vi "Seg1_Charging_Limit_Voltage_checking.vi"(8 "error in (no error)":errorcluster, 9 "Numeric":i32, 10 "Stop Voltage(V)":dbl=4.34 format="%_3f", 11 "VISA Refnum in":refnum<visa-resource-name>) -> (0 "error out":errorcluster, 1 "Boolean":bool, 2 "Voltage Tracking":dbl format="%.8f", 3 "VISA Refnum out":refnum<visa-resource-name>, 5 "Current Tracking":dbl format="%.8f")   [LabVIEW 2015]
uses:
  <instrlib>/Agilent N6700 Series/Agilent N6700 Series.lvlib
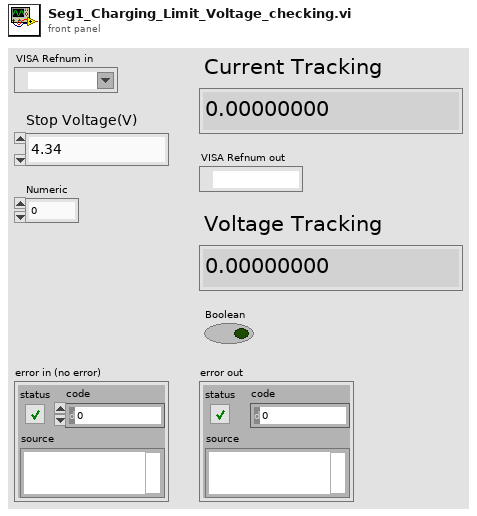
[diagram p1: front panel]
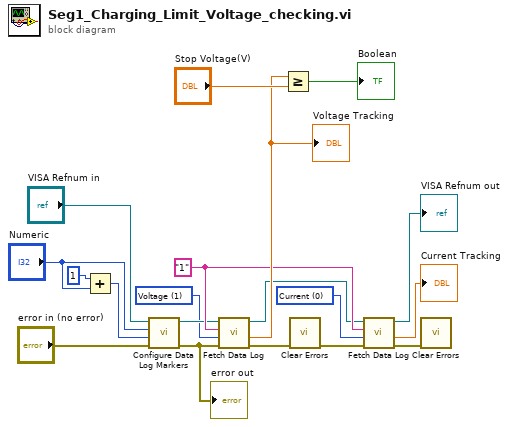
[diagram p0: block diagram]
diagram:
  w10 = 0 items=["Voltage"=1, "Current"=0] ("Data Log Type (1: Voltage)")
  w5 = 1 items=["Voltage"=1, "Current"=0] ("Data Log Type (1: Voltage)")
  w9 = "1" ("Channel Name (1)")
  n1 = Add(x=1, y="Numeric") -> (x+y=w3:i32)
  n2 = call <instrlib>:"Configure Data Log Markers.vi"("error in (no error)"="error in (no error)", "Data Log Marker 2 (27.5 s)"=w3, "Data Log Marker 1 (7.5 s)"="Numeric", "VISA resource name"="VISA Refnum in") -> ("error out"=w16:errorcluster, "VISA resource name out"=w6:refnum<visa-resource-name>)  [unwired: 6 in]
  "error out" <- w16
  n3 = call <instrlib>:"Fetch Data Log.vi"("error in (no error)"=w16, "Data Log Type (1: Voltage)"=w5, "Channel Name (1)"=w9, "VISA resource name"=w6) -> ("error out"=w11:errorcluster, "Peak to Peak"=w14:dbl, "VISA resource name out"=w8:refnum<visa-resource-name>)  [unwired: 5 in]
  "Voltage Tracking" <- w14
  n4 = Greater Or Equal?(x=w14, y="Stop Voltage(V)") -> (x >= y?=→"Boolean":bool)
  n5 = call <vilib>:"Clear Errors.vi"("error in (no error)"=w11) -> ("error out"=w2:errorcluster)  [unwired: 5 in, 1 out]
  n6 = call <instrlib>:"Fetch Data Log.vi"("error in (no error)"=w2, "Data Log Type (1: Voltage)"=w10, "Channel Name (1)"=w9, "VISA resource name"=w8) -> ("error out"=w1:errorcluster, "Peak to Peak"=→"Current Tracking":dbl, "VISA resource name out"=→"VISA Refnum out":refnum<visa-resource-name>)  [unwired: 5 in]
  n7 = call <vilib>:"Clear Errors.vi"("error in (no error)"=w1) -> ()  [unwired: 5 in, 2 out]
